vi "dT-SR810,dP-ADC,withoutT.vi"() -> ()   [LabVIEW 2014]
uses:
  Instance          11 26Saved   Pressure_statistic .vi
  Instance           2 26Saved   Pressure_statistic .vi
  Instance           9 26Saved   Pressure_statistic .vi
  Instance           8 26Saved   Pressure_statistic .vi
  <instrlib>/Stanford Research 830/Public/Data/Read (Multiple Points).vi
  Instance          16 26Saved   Pressure_statistic .vi
  <vilib>/Utility/file.llb/Write To Spreadsheet File (DBL).vi
  <instrlib>/Stanford Research 830/Stanford Research 830.lvlib
panel:
  out "?":sgl[](graph)
  in  "Channel 1 Display (0: X)":u16(ring) items=["X", "R", "X Noise", "Aux In 1", "Aux In 2"]
  in  "Internal Reference Frequency (1000 Hz)":dbl=1000.0
  in  "Sine Output Amplitude (1 V)":dbl=1.0
  in  "Reference Source (1: Internal)":u16(ring)=1 items=["External", "Internal"]
  in  "Input Coupling (0: AC)":u16(ring) items=["AC", "DC"]
  in  "Input Connection (0: Single-Ended Voltage)":u16(ring) items=["Single-Ended Voltage", "Differential Voltage", "1 MOhm Current Gain", "100 MOhm Current Gain"]
  in  "VISA resource name":refnum<visa-resource-name>
  in  "Number of Points (100)":u32=100
  in  "Sample Rate (10: 64 Hz)":u16(ring)=10 items=["62.5 mHz", "125 mHz", "250 mHz", "500 mHz", "1 Hz", "2 Hz", "4 Hz", "8Hz", "16 Hz", "32 Hz", "64 Hz", "128 Hz", "256 Hz", "512 Hz", "Trigger "]
  in  "mkv per degree(thermocouple type)":dbl
  out "T,C":dbl
  out "T,K":dbl
  in  "Tkomn, C":dbl
  in  "Temperature":dbl
  in  "Filter 2":bool
  in  "Case Constant\n(See Context Help)":bool=TRUE
  in  "Write":bool
  out "P, V":dbl[](array[numeric])
  out "Waveform Graph":dynamicdata(graph)
  in  "Fourier transform":bool
  out "Pressure Frequency":dbl
  out "Pressure Amplitude":dbl
  in  "stop":bool
  # "Responce"
  # "Pressure"
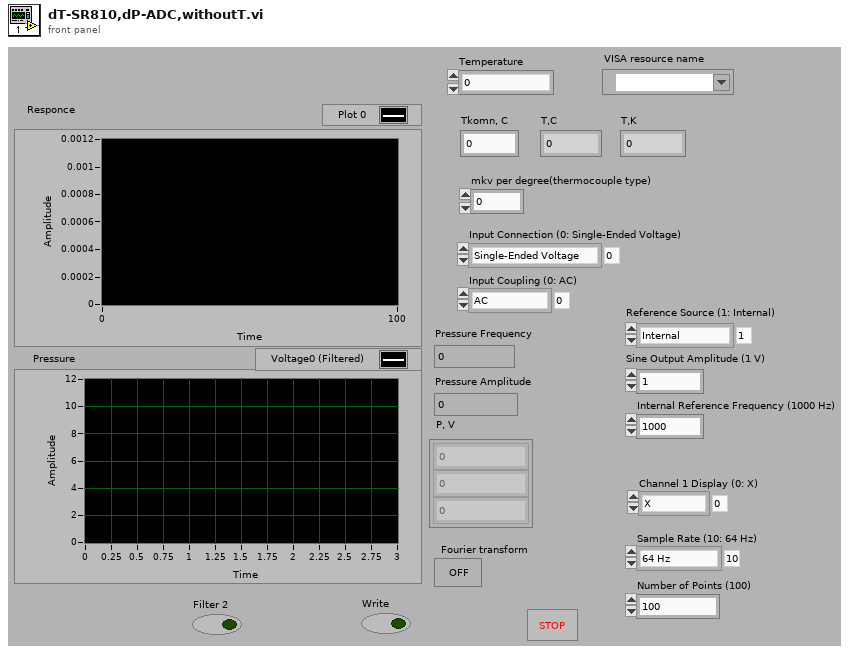
[diagram p1: front panel]
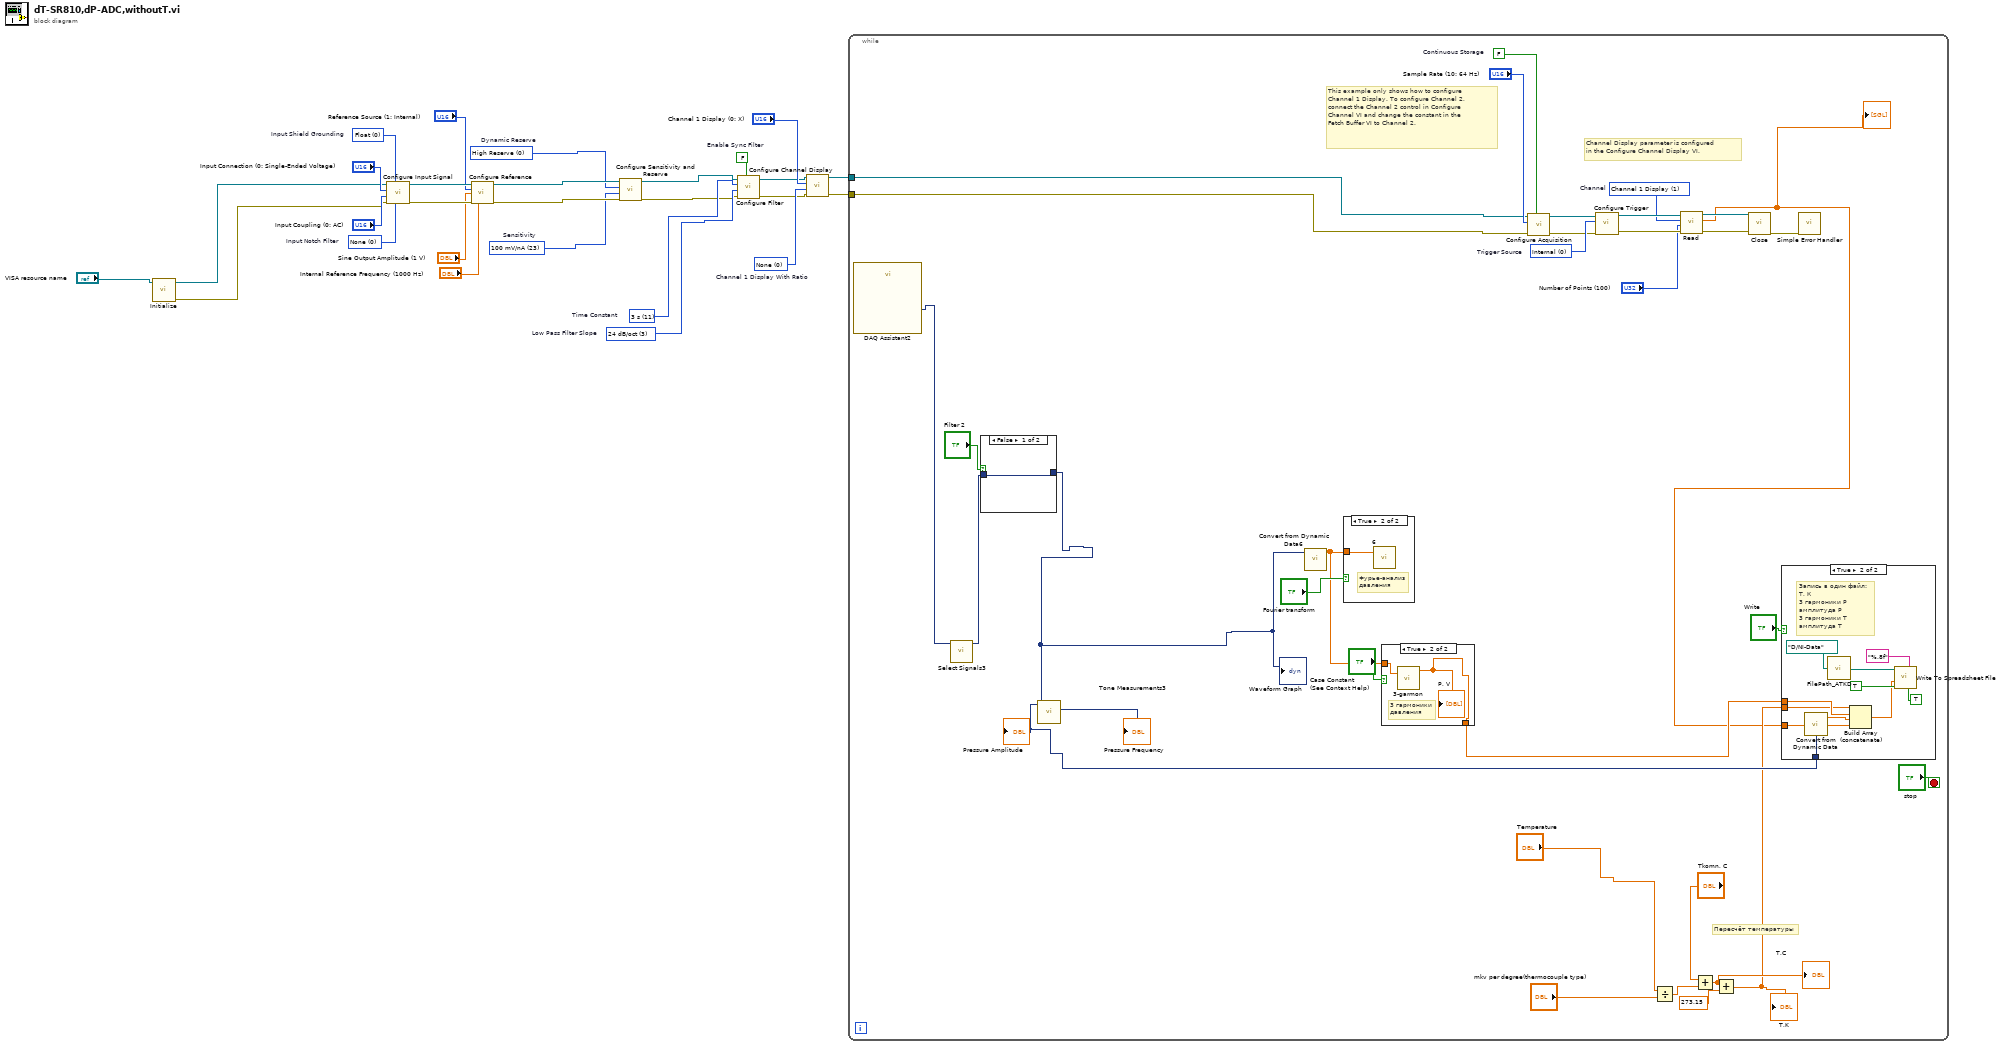
[diagram p0: block diagram]
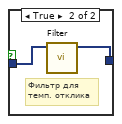
[diagram p2: hidden frame]
diagram:
  w5 = u16 0 items=["None", "Aux In 1", "Aux In 2"]  # Channel 1 Display With Ratio
  w11 = FALSE  # Enable Sync Filter
  w10 = u16 3 items=["6 dB/oct", "12 dB/oct", "18 db/oct", "24 dB/oct"]  # Low Pass Filter Slope
  w9 = u16 11 items=["10 us", "30 us", "100 us", "300 us", "1 ms", "3 ms", "10 ms", "30 ms", "100 ms", "300 ms", "1 s", "3 s", "10 s", "30 s", "100 s", "300 s", "1 ks", "3 ks", "10 ks", "30 ks"]  # Time Constant
  w12 = i16 23 items=["Auto Gain"=-1, "2 nV/fA"=0, "5 nV/fA"=1, "10 nV/fA"=2, "20 nV/fA"=3, "50 nV/fA"=4, "100 nV/fA"=5, "200 nV/fA"=6, "500 nV/fA"=7, "1 uV/pA"=8, "2 uV/pA"=9, "5 uV/pA"=10, "10 uV/pA"=11, "20 uV/pA"=12, "50 uV/pA"=13, "100 uV/pA"=14, "200 uV/pA"=15, "500 uV/pA"=16, "1 mV/nA"=17, "2 mV/nA"=18, "5 mV/nA"=19, "10 mV/nA"=20, "20 mV/nA"=21, "50 mV/nA"=22, "100 mV/nA"=23, "200 mV/nA"=24, "500 mV/mA"=25, "1 V/uA"=26]  # Sensitivity
  w13 = i16 0 items=["Auto Reserve"=-1, "High Reserve"=0, "Normal"=1, "Low Noise"=2]  # Dynamic Reserve
  w21 = u16 0 items=["None", "Line Notch", "2x Line Notch", "Both Notch Filters"]  # Input Notch Filter
  w24 = u16 0 items=["Float", "Ground"]  # Input Shield Grounding
  n1 = call "Initialize.vi"("VISA resource name"="VISA resource name") -> ("error out"=w16:errorcluster, "VISA resource name out"=w17:refnum<visa-resource-name>)  [unwired: 9 in]
  n2 = call "Configure Input Signal.vi"("Input Notch Filter (0: None)"=w21, "Input Shield Grounding (0: Float)"=w24, "error in (no error)"=w16, "Input Coupling (0: AC)"="Input Coupling (0: AC)", "Input Connection (0: Single-Ended Voltage)"="Input Connection (0: Single-Ended Voltage)", "VISA resource name"=w17) -> ("error out"=w25:errorcluster, "VISA resource name out"=w26:refnum<visa-resource-name>)  [unwired: 4 in]
  n3 = call "Configure Reference.vi"("VISA resource name"=w26, "Reference Source (1: Internal)"="Reference Source (1: Internal)", "Sine Output Amplitude (1 V)"="Sine Output Amplitude (1 V)", "error in (no error)"=w25, "Internal Reference Frequency (1000 Hz)"="Internal Reference Frequency (1000 Hz)") -> ("VISA resource name out"=w15:refnum<visa-resource-name>, "error out"=w14:errorcluster)  [unwired: 9 in]
  n4 = call "Configure Sensitivity and Reserve.vi"("error in (no error)"=w14, "Sensitivity (-1: Auto gain)"=w12, "Dynamic Reserve (-1: Auto Reserve)"=w13, "VISA resource name"=w15) -> ("error out"=w7:errorcluster, "VISA resource name out"=w8:refnum<visa-resource-name>)  [unwired: 6 in]
  n5 = call "Configure Filter.vi"("Enable Sync Filter (F: Disable)"=w11, "error in (no error)"=w7, "Low Pass Filter Slope (1: 12dB/oct)"=w10, "Time Constant (8: 100ms)"=w9, "VISA resource name"=w8) -> ("error out"=w3:errorcluster, "VISA resource name out"=w4:refnum<visa-resource-name>)  [unwired: 5 in]
  n6 = call "Configure Channel Display.vi"("error in (no error)"=w3, "Channel 1 Display With Ratio (0: None)"=w5, "Channel 1 Display (0: X)"="Channel 1 Display (0: X)", "VISA resource name"=w4) -> ("error out"=w1:errorcluster, "VISA resource name out"=w2:refnum<visa-resource-name>)  [unwired: 6 in]
  n7 = while {
    tunnel: w2 -> [w31]
    tunnel: w1 -> [w30]
    stop <- "stop" stop-if-true
    w33 = u16 1 items=["Channel 1 Display"=1, "Channel 2 Display"=2]  # Channel
    w42 = u16 0 items=["Internal", "External"]  # Trigger Source
    w40 = FALSE  # Continuous Storage
    # "Channel Display parameter is configured\nin the Configure Channel Display VI."
    # "This example only shows how to configure Channel 1 Display. To configure Channel 2, connect the Channel 2 control in Configure Channel VI and change the constant in the Fetch Buffer VI to Channel 2."
    # "Пересчёт температуры"
    n8 = call "DAQ Assistant2"() -> ("data"=w58:dynamicdata)  [unwired: 2 in, 9 out]
    n9 = call "Select Signals3"("Signals"=w58) -> ("Signal Out"=w52:dynamicdata)  [unwired: 1 in, 9 out]
    n10 = case shown="False" "Filter 2" {
      tunnel: w52 -> [w62 w64]
      tunnel: [w62 w63] -> w50
      frame False {
      }
      frame True {
        # "Фильтр для\nтемп. отклика"
        n11 = call "Filter"("Signal"=w64) -> ("Filtered Signal"=w63:dynamicdata)  [unwired: 2 in, 8 out]
      }
    }
    "Waveform Graph" <- w50
    n12 = call "Tone Measurements3"("Signals"=w50) -> ("Frequency"=→"Pressure Frequency":dynamicdata, "Amplitude"=w53:dynamicdata)  [unwired: 1 in, 8 out]
    "Pressure Amplitude" <- w53
    n13 = call "Convert from Dynamic Data6"("Dynamic Data Type"=w50) -> ("Array"=w55:dbl[])  [unwired: 3 out]
    n14 = case shown="True" "Fourier transform" {
      tunnel: w55 -> [_ w78]
      frame False {
      }
      frame True {
        # "Фурье-анализ\nдавления"
        n15 = call "6.vi"("X"=w78) -> ()  [unwired: 7 out]
      }
    }
    n16 = case shown="True" "Case Constant\n(See Context Help)" {
      tunnel: w55 -> [_ w77]
      tunnel: [_ w76] -> w54
      frame False {
      }
      frame True {
        # "3 гармоники\nдавления"
        n17 = call "3-garmon.vi"("X"=w77) -> ("A"=w76:dbl[])  [unwired: 6 out]
        "P, V" <- w76
      }
    }
    n18 = call "Configure Acquisition.vi"("Continuous Storage (T: Enable)"=w40, "error in (no error)"=w30, "Sample Rate (0: 62.5 mHz)"="Sample Rate (10: 64 Hz)", "VISA resource name"=w31) -> ("error out"=w38:errorcluster, "VISA resource name out"=w39:refnum<visa-resource-name>)  [unwired: 6 in]
    n19 = call "Configure Trigger.vi"("error in (no error)"=w38, "Trigger Source (0: Internal)"=w42, "VISA resource name"=w39) -> ("error out"=w36:errorcluster, "VISA resource name out"=w37:refnum<visa-resource-name>)  [unwired: 7 in]
    n20 = Divide(x="Temperature", y="mkv per degree(thermocouple type)") -> (x/y=w48:dbl)
    n21 = call-poly <instrlib>:"Read.vi"("error in (no error)"=w36, "Number of Points (100)"="Number of Points (100)", "Channel (1: Channel 1 Display)"=w33, "VISA resource name"=w37) -> ("error out"=w34:errorcluster, "Measurements"=w28:sgl[], "VISA resource name out"=w35:refnum<visa-resource-name>)  [unwired: 5 in]
    "?" <- w28
    n22 = Add(x="Tkomn, C", y=w48) -> (x+y=w46:dbl)
    "T,C" <- w46
    n23 = Add(x=w46, y=273.15) -> (x+y=w44:dbl)
    "T,K" <- w44
    n24 = call "Close.vi"("error in (no error)"=w34, "VISA resource name"=w35) -> ("error out"=w43:errorcluster)  [unwired: 9 in]
    n25 = case shown="True" "Write" {
      tunnel: w54 -> [_ w75]
      tunnel: w53 -> [_ w69]
      tunnel: w44 -> [_ w66]
      tunnel: w28 -> [_ w65]
      frame False {
      }
      frame True {
        # "Запись в один файл:\nТ, К\n3 гармоники P\nамплитуда P\n3 гармоники Т\nамплитуда Т"
        n26 = call "Convert from Dynamic Data"("Dynamic Data Type"=w69) -> ("Array"=w68:dbl[])  [unwired: 3 out]
        n27 = call "FilePath_ATKD.vi"("base folder path"=path "D:/NI-Data") -> ("ATKD"=w74:path)  [unwired: 3 out]
        n28 = Build Array (concatenate)(w66, w75, w68, w65) -> (w67:dbl[])
        n29 = call-poly <vilib>:"Write To Spreadsheet File.vi"("transpose? (no:F)"=TRUE, "format (%.3f)"="%.8f", "append to file? (new file:F)"=TRUE, "1D data"=w67, "file path (dialog if empty)"=w74) -> ()  [unwired: 1 in, 3 out]
      }
    }
    n30 = call <vilib>:"Simple Error Handler.vi"("error in (no error)"=w43) -> ()  [unwired: 4 in, 5 out]
  }
